vi "get_plot_data.vi"(8 "error in (no error)":errorcluster, 10 "PrepLineObjectName":string) -> (0 "error out":errorcluster, 2 "value history":cluster{"time as number":dbl, "Value":dbl}[](array[cluster]))   [LabVIEW 2015]
doc: "returns the value-history data of the given \"PrepLineObject\". Can be used to greate the history plot"
uses:
  Classes/PrepLineObject/PrepLineObject.lvclass
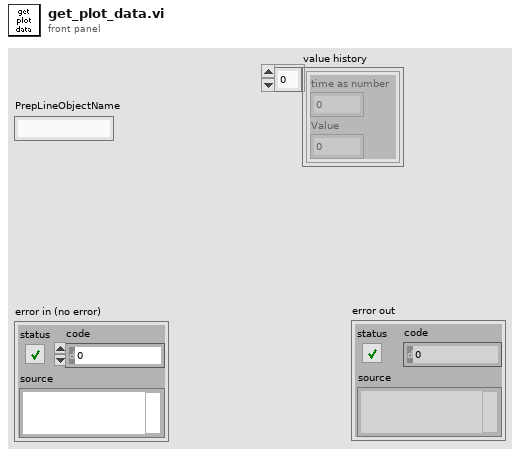
[diagram p1: front panel]
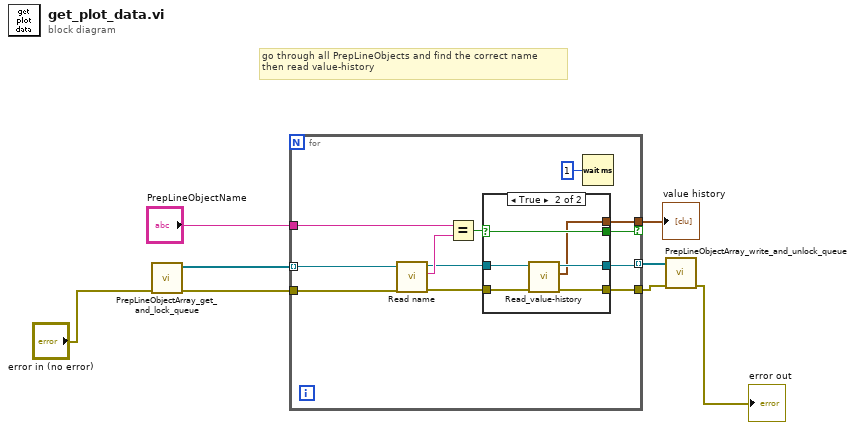
[diagram p0: block diagram]
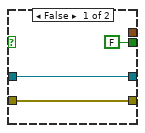
[diagram p2: hidden frame]
diagram:
  # "go through all PrepLineObjects and find the correct name\nthen read value-history"
  n1 = call "PrepLineObjectArray_get_and_lock_queue.vi"("error in (no error)"="error in (no error)") -> ("error out"=w1:errorcluster, "PrepLineObjects"=w6:refnum<class "PrepLineObject.lvclass">[])  [unwired: 9 in]
  n2 = for {
    tunnel: w6 -> [w18] mode=indexing
    tunnel: "PrepLineObjectName" -> [w19]
    tunnel: [w9] -> w7 if=w15
    tunnel: [w12] -> w5 mode=indexing
    tunnel: [w11] -> w4
    tunnel: w1 -> [w10]
    n3 = call-dynamic "Read name.vi"("error in (no error)"=w10, "PrepLineObject in"=w18) -> ("error out"=w13:errorcluster, "name"=w20:string, "PrepLineObject out"=w14:refnum<class "PrepLineObject.lvclass">)  [unwired: 7 in]
    n4 = Equal?(x=w19, y=w20) -> (x = y?=w16:bool)
    n5 = case shown="True" w16 {
      selector: w16 -> [_ w29]
      tunnel: [FALSE w29] -> w15
      tunnel: w14 -> [w23 w28]
      tunnel: w13 -> [w22 w27]
      tunnel: [w23 w26] -> w12
      tunnel: [w22 w25] -> w11
      tunnel: [_ w24] -> w9
      frame False {
      }
      frame True {
        n6 = call-dynamic "Read_value-history.vi"("error in (no error)"=w27, "PrepLineObject in"=w28) -> ("error out"=w25:errorcluster, "value history"=w24:cluster{"time as number":dbl, "Value":dbl}[], "PrepLineObject out"=w26:refnum<class "PrepLineObject.lvclass">)  [unwired: 7 in]
      }
    }
    n7 = Wait (ms)(milliseconds to wait=u32 1) -> ()  [unwired: 1 out]
  }
  "value history" <- w7
  n8 = call "PrepLineObjectArray_write_and_unlock_queue.vi"("error in (no error)"=w4, "PrepLineObjArray"=w5) -> ("error out"=→"error out":errorcluster)  [unwired: 9 in]
